vi "Untitled 1.vi"() -> ()   [LabVIEW 2018]
panel:
  out "Image":T1(plugin-control)
  out "error out":errorcluster
  in  "error in (no error)":errorcluster
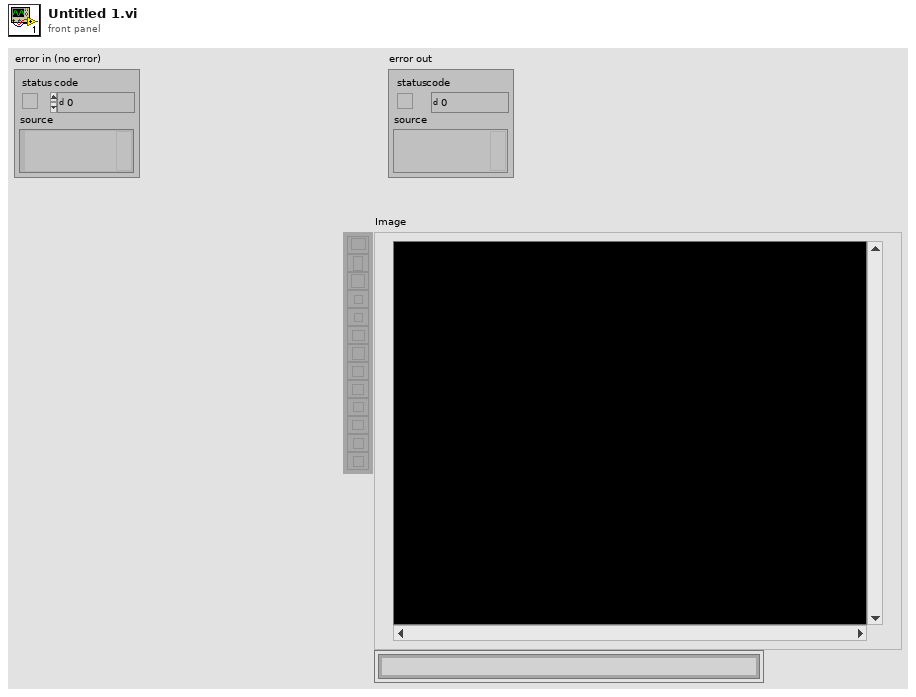
[diagram p1: front panel]
types:
  T1 = typedef "IMAQ Image.ctl" = refnum<image>
  T2 = typedef "Image Type" = u32
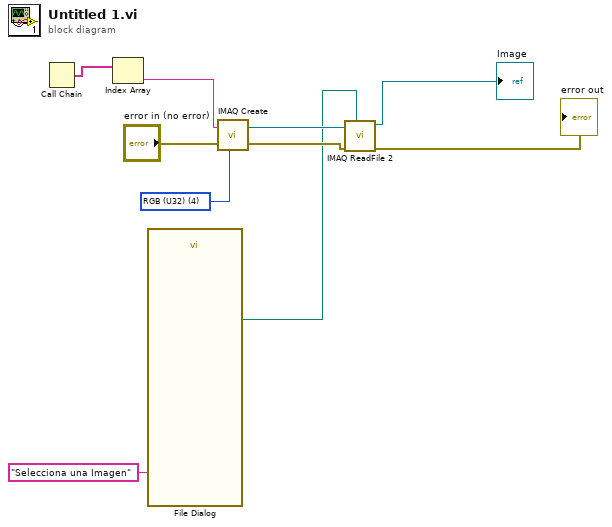
[diagram p0: block diagram]
diagram:
  w2 = T2 4 items=["Grayscale (U8)", "Grayscale (I16)", "Grayscale (SGL)", "Complex (CSG)", "RGB (U32)", "HSL (U32)", "RGB (U64)", "Grayscale (U16)"] ("Image Type")
  n1 = Call Chain() -> (call chain=w10:string[])
  n2 = Index Array(array=w10) -> (element=w8:string)  [unwired: 1 in]
  n3 = call "File Dialog"("prompt"="Selecciona una Imagen") -> ("selected path"=w1:path)  [unwired: 11 in, 3 out]
  n4 = call "IMAQ Create"("Image Name"=w8, "Image Type"=w2, "error in (no error)"="error in (no error)") -> ("New Image"=w3:T1, "error out"=w9:errorcluster)  [unwired: 2 in]
  n5 = call "IMAQ ReadFile 2"("File Path"=w1, "error in (no error)"=w9, "Image"=w3) -> ("error out"=→"error out":errorcluster, "Image Out"=→"Image":T1)  [unwired: 4 in, 3 out]
